vi "10-Tap 8-Bit Camera with DRAM (Host).vi"() -> ()   [LabVIEW 2018]
doc: "This is the host VI for the 10-Tap 8-Bit Camera with DRAM example. This example demonstrates how to acquire images from a 10-tap, 8-bit, extended configuration, Camera Link camera and display the images on the host. This example supports area scan and line scan cameras for both continuous and finite acquisitions.\n\nThis example also demonstrates the use of DRAM as a frame buffer for very high speed acquisitions. Data packing and flow-control are also employed to maximize use of the available DRAM and FIFOs in terms of both memory space and performance.\n\nAdditionally, the example demonstrates the serial server, which allows third-party camera configuration utilities to communicate with the camera using the Camera Link serial interface while this VI is running."
uses:
  <vilib>/userdefined/High Color/nirio_resource_hc.ctl
  <vilib>/Analysis/Matrix/Datatypes/RealMatrix.ctl
  <vilib>/Platform/TimedLoop/XDataNode/timing_clust.ctl
  <vilib>/Platform/TimedLoop/XDataNode/nitl_modes.ctl
  <vilib>/Platform/TimedLoop/XDataNode/wakeup.ctl
  <vilib>/DAQmx/write.llb/DAQmx Write (Analog DBL 1Chan 1Samp).vi
  <vilib>/Analysis/baseanly.llb/Real A x B.vi
  <vilib>/FPGAPlugInAG/PCIe-1473R/niLvFpga_Open_PCIe-1473R.vi
  <vilib>/rvi/interface/common/dynamic/niFpgaDynamicAddResources.vi
  <vilib>/FPGAPlugInAG/Dynamic/niLvFpga_Reset_Dynamic.vi
  <vilib>/Analysis/Matrix/Numeric/Conversions/Array To Matrix - RA2.vi
  <userlib>/DAQNavi Polymorphic VI/create/DAQNavi Create Channel(CI-UpDown Count Value).vi
  <vilib>/Utility/error.llb/Error Cluster From Error Code.vi
  <vilib>/rvi/errors/niLvFpgaAdjustHostInterfaceError.vi
  <vilib>/FPGAPlugInAG/Dynamic/niLvFpga_Run_Dynamic.vi
  <vilib>/rvi/interface/common/niFpgaWaitOnOcc.vi
  <userlib>/DAQNavi Polymorphic VI/read/DAQNavi Read (Counter Count Value 1Chan 1Samp).vi
  <vilib>/Analysis/Matrix/Numeric/Conversions/Array To Matrix - RA.vi
  <vilib>/Analysis/Matrix/Numeric/Conversions/Matrix To Array - RM.vi
  <vilib>/DAQmx/miscellaneous.llb/DAQmx Fill In Error Info.vi
  <vilib>/FPGAPlugInAG/Dynamic/niLvFpga_Close_Dynamic.vi
  <vilib>/platform/TimedLoop/XDataNode/XDataNode.xnode
  <vilib>/rvi/interface/nirviOpenFPGA/nirviOpenFPGA.xnode
  FPGA Bitfiles/10-Tap8-bitCamer_FPGATarget_10-Tap8-bitCamer_C490DC32.lvbitx
  <vilib>/rvi/interface/nirviMethod/nirviMethod.xnode
  <vilib>/rvi/interface/nirviReadWriteControl/nirviReadWriteControl.xnode
  <vilib>/rvi/interface/nirviCloseFPGA/nirviCloseFPGA.xnode
  <vilib>/rvi/interface/Simulation/niFpgaSimulationCallBeginRW.vi
  <vilib>/rvi/errors/niLvFpgaMergeErrorWithErrorCode.vi
  NiFpgaLv.dll
  <vilib>/FPGAPlugInAG/Dynamic/niLvFpga_ConfigureFifo_Dynamic.vi
  <vilib>/FPGAPlugInAG/Dynamic/niLvFpga_StartFifo_Dynamic.vi
  <vilib>/FPGAPlugInAG/Dynamic/niLvFpga_ReadFifo_Dynamic.vi
  <vilib>/Platform/TimedLoop/XDataNode/XDNodeRunTimeDep.lvlib
  <resource>/objmgr/ni.dex.rc
  MPC_dll_4_vs17_cv3_4/x64/Release/MPC_dll_4_vs17_cv3_4.dll
  <vilib>/ErrorRing/Error Ring.xnode
  <vilib>/Analysis/NI_AALBase.lvlib
  <vilib>/Analysis/Matrix/NI_Matrix.lvlib
  fish tracking dll vc17 opencv3_4/x64/Release/fish tracking dll vc17 opencv3_4.dll
panel:
  in  "length_fish":i32=115
  in  "width_fish":i32=20
  in  "ROI_height":i32=110
  in  "ROI_witdth":i32=110
  in  "Object Threshold":i32=200
  in  "BinThreshold":i32=100
  in  "Templates size":i32=48
  in  "shift_head2yolk":i32=30
  in  "address":string="192.168.1.27"
  out "# elements in queue 2":i32
  out "Numeric":i32
  out "concatenated string":string
  out "bytes written":i32
  in  "shift":i32=9
  in  "gamma":dbl=0.04 format="%#_13g"
  out "Cluster":cluster{"data":i32, i32}
  out "Real Matrix 5":T1
  out "Real Matrix 4":T1
  out "Real Matrix 2":T1
  out "Real Matrix":T1
  out "A x B 2":T1
  out "A x B":T1
  out "error out":errorcluster
  in  "send":bool
  out "Is Connected":bool
  in  "update ratio":dbl=0.1
  in  "Start Serial Server":bool=TRUE
  in  "Stopped 2":bool
  in  "display":bool
  out "Image":T2(plugin-control)
  in  "reset 2":bool
  in  "reset frame":bool
  in  "reset position":bool
  out "max load a frame":dbl
  out "max load a position":dbl
  out "# elements in queue":i32
  out "element":dbl[](array[numeric])
  in  "start sending":bool
  out "connected":bool
  in  "Acquire":bool
  out "max distance 2":i32
  out "out of FOV 2":i32
  in  "count":bool
  out "max distance":i32
  out "out of FOV":i32
  out "Stage Position Y":i32=520
  out "Stage Position X":i32=520
  out "#timeout3":i32
  out "#timeout1":i32
  out "max time4 image and position loading":dbl
  out "max time3 total":dbl
  out "max time2 detection":dbl
  out "max time1 detection+command":dbl
  out "time loading a frame":dbl
  in  "length of fish_history":i32=4
  in  "m(length of kernel)":i32=30
  out "Heading":cluster{dbl, dbl}
  out "process":i32
  in  "Target Y":i32(slide)=177 min=0 max=384 scale=130.0..230.0
  in  "Target X":i32(slide)=198 min=0 max=520 scale=130.0..230.0
  out "y":dbl
  out "x":dbl
  in  "Controller":picture
  out "Y Resolution":i32
  out "X Resolution":i32
  in  "Track":bool
  out "Frame #":i32=72
  out "电压2":dbl
  out "电压1":dbl
  out "fish FOUND":bool
  out "Centroid":cluster{"x":i32, "y":i32}
  out "TimeDelay":dbl
  in  "DMA Buffer Size\n(In Images)":u32=64 caption="DMA Buffer Size"
  in  "Signal Mapping":T3(ring)=enum."Basler 10-tap"
  out "Acq In Progress":bool
  in  "Line Scan":bool
  in  "Cancel":bool
  out "Acq'd Frame Width":u32
  in  "Stopped":bool
  in  "RIO Device":T4="RIO0"
  out "DMA Write Timeout":bool
  out "Frames Acq'd":u32
  out "Acq'd Frame Height":u32
  in  "Stop":bool
  in  "Image Height":u32=360 max=65535
  in  "Image Width":u32=360 max=65535 step=40
  out "Initialized":bool
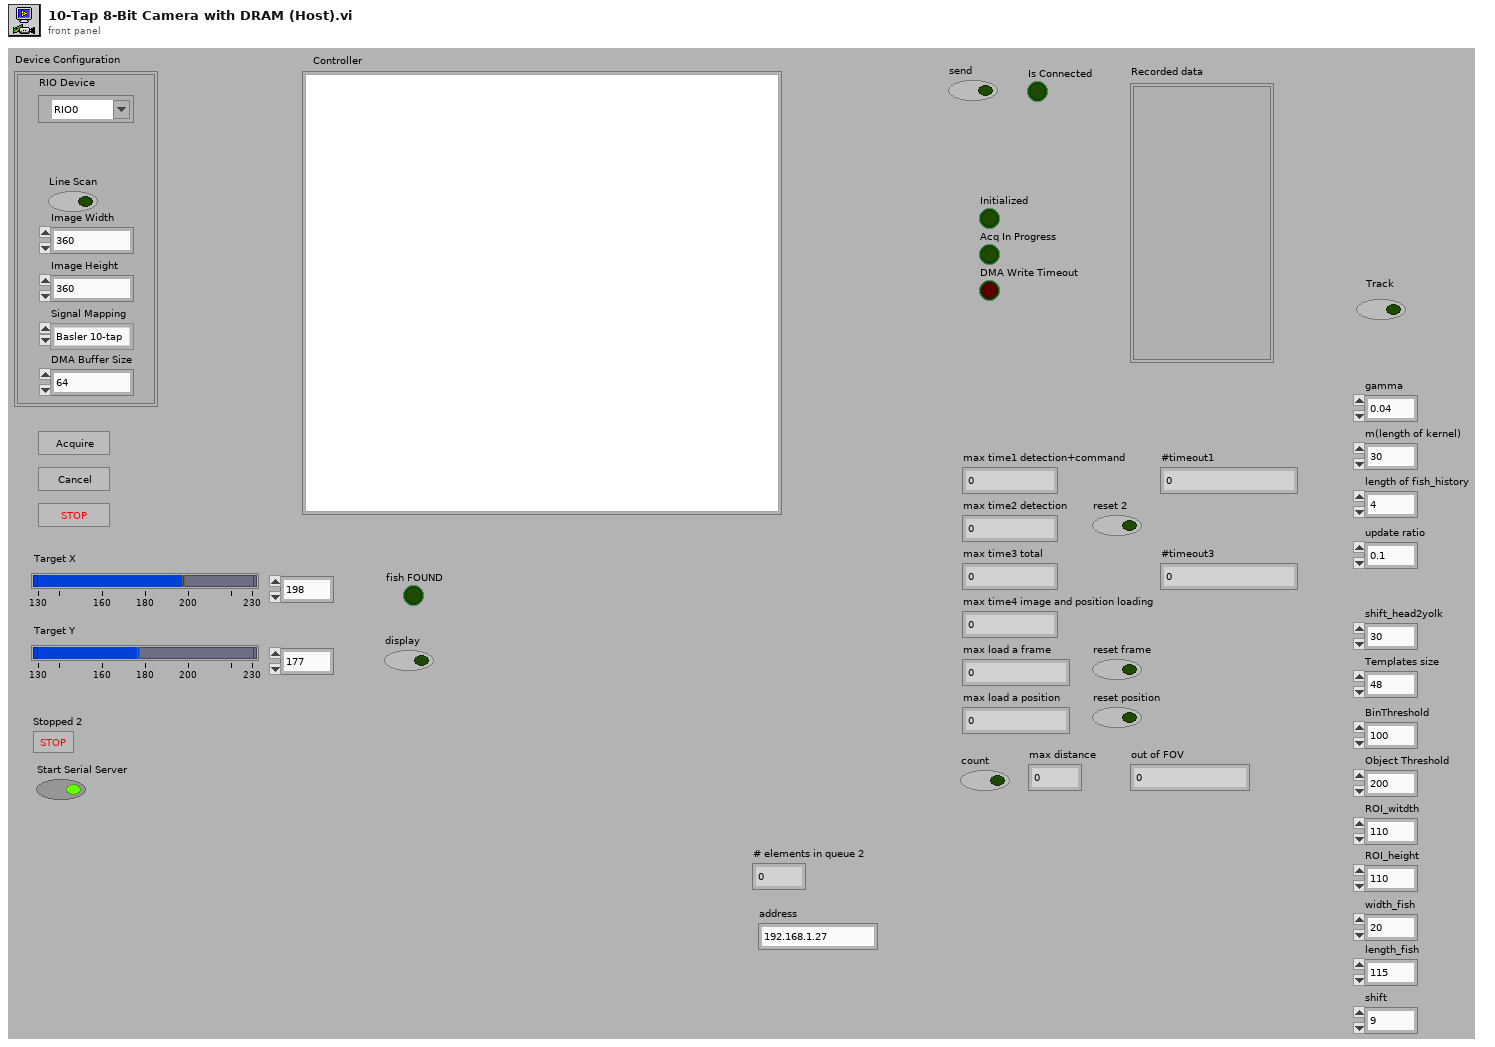
[diagram p1: front panel]
types:
  T1 = typedef "NI_Matrix.lvlib/RealMatrix.ctl" = dbl[][]
  T2 = typedef "IMAQ Image.ctl" = refnum<image>
  T3 = enum8{"Standard", "Basler 10-tap", "Vosskühler 10-tap"}
  T4 = typedef "nirio_resource_hc.ctl" = tag
  T5 = typedef "Image Type" = u32
  T6 = typedef "XDNodeRunTimeDep.lvlib/timing_clust.ctl" = cluster{"Expected End [f-1]":u64, "Actual End [f-1]":u64, "Finished Late? [f-1]":bool, "Expected End [i-1]":u64, "Actual End [i-1]":u64, "Finished Late? [i-1]":bool, "Expected Start [i]":u64, "Actual Start [i]":u64, "Expected Start [f]":u64, "Actual Start [f]":u64, "Source Name":string, "Structure Name":string, "Period":i64, "Deadline":i64, "Offset":i64, "Start":i64, "Priority":i32, "Timeout":i32, "Mode":T7, "Wakeup Reason":T8, "Error":errorcluster, "Source Type":string, "Secondary Source Type":string, "Global End Time":u64, "Global Start Time":u64, "Frame Duration":u64, "Iteration Duration":u64, "Assigned CPU":i32, "I/O Scan Engine Mode":u32}
  T7 = typedef "XDNodeRunTimeDep.lvlib/nitl_modes.ctl" = enum32{"No Change", "Process missed periods, maintain original phase", "Discard missed periods, maintain original phase", "Process missed periods, ignore original phase", "Discard missed periods, ignore original phase"}
  T8 = typedef "XDNodeRunTimeDep.lvlib/wakeup.ctl" = enum32{"Normal", "Aborted", "Asynchronous wakeup", "Timing source error", "Timed loop error", "Timeout"}
  T9 = enum16{"big-endian, network order", "native, host order", "little-endian"}
  T10 = typedef "LVPoint32TypeDef.ctl" = cluster{"Horizontal":i32, "Vertical":i32}
  T11 = typedef "LVPositionTypeDef.ctl" = cluster{"Left":i32, "Top":i32}
  T12 = typedef "LVBoundsTypeDef.ctl" = cluster{"Width":u32, "Height":u32}
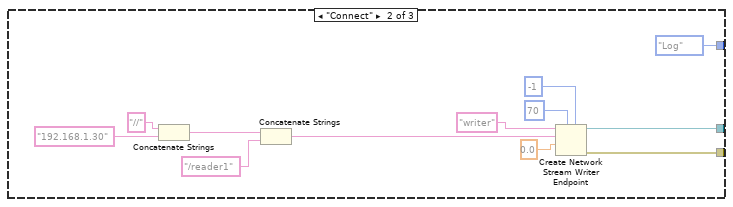
[diagram p4: hidden frame]
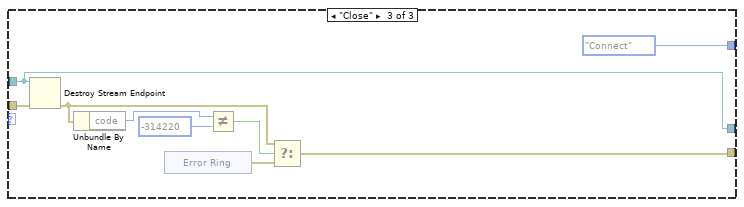
[diagram p5: hidden frame]
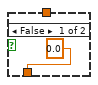
[diagram p13: hidden frame]
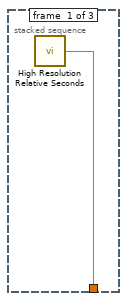
[diagram p14: hidden frame]
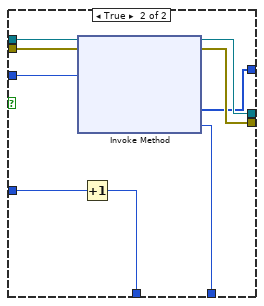
[diagram p15: hidden frame]
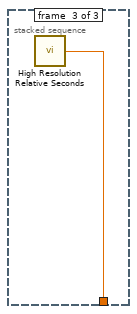
[diagram p16: hidden frame]
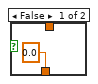
[diagram p17: hidden frame]
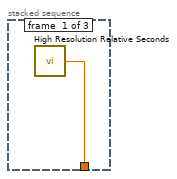
[diagram p18: hidden frame]
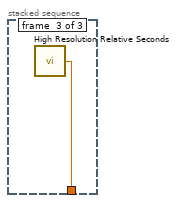
[diagram p19: hidden frame]
diagram:
  w38 = 72 ("n_templates")
  w40 = 0
  w61 = 2
  w55 = 0
  w62 = 0.0
  w86 = T5 0 items=["Grayscale (U8)", "Grayscale (I16)", "Grayscale (SGL)", "Complex (CSG)", "RGB (U32)", "HSL (U32)", "RGB (U64)", "Grayscale (U16)"] ("Image Type")
  w100 = refnum<k21> "Stage_Y"  # DAQmx任务名
  w101 = refnum<k21> "Stage_X"  # DAQmx任务名
  w103 = T5 0 items=["Grayscale (U8)", "Grayscale (I16)", "Grayscale (SGL)", "Complex (CSG)", "RGB (U32)", "HSL (U32)", "RGB (U64)", "Grayscale (U16)"] ("Image Type")
  w109 = u32 8  # Pixels per DMA word
  w140 = T5 0 items=["Grayscale (U8)", "Grayscale (I16)", "Grayscale (SGL)", "Complex (CSG)", "RGB (U32)", "HSL (U32)", "RGB (U64)", "Grayscale (U16)"] ("Image Type")
  # "Start the Serial Server to allow serial communication\nwith the camera. This allows third-party camera\nconfiguration utilites to be used."
  # "If your camera outputs active-low enable\nsignals or does not use DVAL then you \ncan change the configuration here."
  # "Configure the DMA FIFO memory buffer to be\nlarge enough for several frames. This provides\nbuffering to help deal with system latencies."
  # "Start running\nthe FPGA VI."
  # "Reset FPGA to clear\nany current state."
  # "Read the specified image\nwidth and height. In this\nexample, these must be set\nbefore starting the VI."
  # "Merge any errors.\nClean up the image.\nClose the FPGA reference.\nDisplay any errors."
  # "Acquire frames as requested.\nUse the width and height to determine how much data to read from the DMA FIFO.\nConvert the data into a Vision Image for display."
  # "Monitor the acquisition status"
  # "Create an image of the type to be displayed."
  # "Initialize the acquisition interface on the FPGA.  This will\nwait until a pixel clock is detected from the camera."
  # "Initialize the DMA FIFO for transferring\ndata from FPGA target to the host."
  # "Configure the Camera Link interface.\nThis needs to be done prior to running\nthe FPGA block diagram."
  # "Open a reference to the FPGA bitstream\nand initialize the user interface."
  n1 = flat-sequence {
    tunnel: [w146] -> w135
    tunnel: [w145] -> w144
    frame #0 {
      w149 = u32 0 ("Num Lines Acq'd")
      w148 = FALSE ("stop")
      n2 = local write "DMA Write Timeout"(w148) -> ()
      n3 = local write "Acq'd Frame Width"(w149) -> ()
      n4 = local write "Acq'd Frame Height"(w149) -> ()
      n5 = local write "Stopped"(w148) -> ()
      n6 = local write "Frames Acq'd"(w149) -> ()
      n7 = local write "Initialized"(w148) -> ()
      n8 = xnode "打开FPGA VI引用句柄"("resource name"="RIO Device") -> ("FPGA VI Reference Out"=w146:refnum<k20>, "error out"=w145:errorcluster)  [unwired: 1 in]
    }
  }
  n9 = xnode "Invoke Method"("FPGA VI Reference In"=w135, "error in"=w144) -> ("FPGA VI Reference Out"=w125:refnum<k20>, "error out"=w127:errorcluster)
  n10 = xnode "Read/Write Control"("FPGA VI Reference In"=w125, "error in"=w127, "CL Config.FVAL Active High"=TRUE ("IO Module Config.CL FVAL Active High"), "CL Config.LVAL Active High"=TRUE ("IO Module Config.CL LVAL Active High"), "CL Config.DVAL Active High"=TRUE ("IO Module Config.CL DVAL Active High"), "CL Config.Spare Active High"=TRUE ("IO Module Config.CL Spare Active High"), "CL Config.Line Scan"="Line Scan", "Acq Control.Ignore DVAL"=FALSE ("CL Config.Line Scan"), "CL Config.Configuration"=enum8{"Base", "Medium", "Full"}."Full", "CL Config.Signal Mapping"="Signal Mapping") -> ("FPGA VI Reference Out"=w128:refnum<k20>, "error out"=w126:errorcluster)
  n11 = xnode "Invoke Method"("FPGA VI Reference In"=w128, "error in"=w126) -> ("FPGA VI Reference Out"=w106:refnum<k20>, "error out"=w105:errorcluster)  [unwired: 1 in]
  n12 = Multiply(x="Image Height", y="Image Width") -> (x*y=w108:u32)
  n13 = Quotient & Remainder(x=w108, y=w109) -> (floor(x/y)=w107:u32)  [unwired: 1 out]
  n14 = Multiply(x=w107, y="DMA Buffer Size\n(In Images)") -> (x*y=w119:u32)
  n15 = xnode "Invoke Method"("FPGA VI Reference In"=w106, "error in"=w105, "请求的深度"=w119) -> ("FPGA VI Reference Out"=w134:refnum<k20>, "error out"=w133:errorcluster)  [unwired: 1 out]
  n16 = xnode "Invoke Method"("FPGA VI Reference In"=w134, "error in"=w133) -> ("FPGA VI Reference Out"=w120:refnum<k20>, "error out"=w132:errorcluster)
  n17 = xnode "读取/写入控件"("FPGA VI Reference In"=w120, "error in"=w132, "Acq Control.Initialize"=TRUE ("Arm Acquisition")) -> ("FPGA VI Reference Out"=w143:refnum<k20>, "error out"=w142:errorcluster)
  n18 = while {
    tunnel: w143 -> [w157]
    tunnel: w142 -> [w156]
    tunnel: [w155] -> w25
    tunnel: [w159] -> w116
    i -> [w151]
    stop <- w162 stop-if-true
    # "A custom error is generated if the acquisition unit has not become\ninitialized within 2 seconds. This typically occurs when a camera is\nnot connected, is not powered, or is not of the correct type."
    n19 = xnode "读取/写入控件"("FPGA VI Reference In"=w157, "error in"=w156) -> ("FPGA VI Reference Out"=w155:refnum<k20>, "error out"=w154:errorcluster, "Acq Status.Initialized"=w153:bool)
    n20 = Wait (ms)(milliseconds to wait=u32 100) -> ()  [unwired: 1 out]
    n21 = Greater?(x=w151, y=20) -> (0:w152:bool)
    n22 = case shown="True" w152 {
      tunnel: [w164 FALSE] -> w158
      tunnel: w153 -> [w164 _]
      tunnel: w154 -> [w163 w166]
      tunnel: [w163 w168] -> w159
      frame False {
      }
      frame True {
        n23 = Merge Errors(w166, errorcluster {"status"=TRUE, "code"=-8999, "source"="Acquisition Initialization: This error typically occurs when a camera is not properly connected, is not powered, or is not of the correct type."} ("error in")) -> (w168:errorcluster)
      }
    }
    "Initialized" <- w158
    n24 = Unbundle By Name(w159) -> ("status"=w161:bool)
    n25 = Or(x=w161, y=w158) -> (x .or. y?=w162:bool)
  }
  n26 = case shown="True" "Start Serial Server" {
    tunnel: [_ w169] -> w24
    tunnel: w25 -> [_ w170]
    frame False {
    }
    frame True {
      n27 = control-ref of="Stopped 2"() -> (w171:refnum<vi>)
      n28 = call "SerialServer.vi"("Stop Refnum"=w171, "FPGA VI Reference In"=w170) -> ("FPGA VI Reference Out"=w169:refnum<k20>)  [unwired: 5 in]
    }
  }
  n29 = call "IMAQ Create"("Image Name"="Image", "Image Type"=w140, "error in (no error)"=w116) -> ("New Image"=w113:T2, "error out"=w112:errorcluster)  [unwired: 2 in]
  n30 = Add(x="length of fish_history", y=1) -> (x+y=w57:i32)
  n31 = Initialize Array(0.0, 7) -> (w27:dbl[])
  n32 = Obtain Queue(max queue size (-1, unlimited)=3, name (unnamed)="tracking result" ("Image Name"), element data type=w27) -> (queue out=w23:refnum<queue>)  [unwired: 2 in, 2 out]
  n33 = Multiply(x=w61, y=w57) -> (x*y=w54:i32)
  n34 = To Unsigned Byte Integer(number=w40) -> (unsigned 8bit integer=w41:u8)
  n35 = Add(x="m(length of kernel)", y=1) -> (x+y=w42:i32)
  n36 = Initialize Array(w41, w40, w40, w40) -> (w39:u8[][][])
  n37 = for {
    N: w38 -> [_]
    shift-right: [w173] -> w37
    shift-left: w39 -> [w174]
    i -> [w172]
    w178 = T5 0 items=["Grayscale (U8)", "Grayscale (I16)", "Grayscale (SGL)", "Complex (CSG)", "RGB (U32)", "HSL (U32)", "RGB (U64)", "Grayscale (U16)"] ("Image Type")
    n38 = Number To Decimal String(number=w172) -> (decimal integer string=w182:string)  [unwired: 1 in]
    n39 = Concatenate Strings(w182, ".jpg") -> (w181:string)
    n40 = Build Path(base path=path "F:/TrackingUsingOpenCV3_with_bkg_subtr_and_pred_and_temp_matching_nodisplay - 210309/templates" ("Templates Path"), name or relative path=w181) -> (appended path=w180:path)
    n41 = call "IMAQ Create"("Image Name"="Temp", "Image Type"=w178) -> ("New Image"=w177:T2)  [unwired: 3 in, 1 out]
    n42 = call "IMAQ ReadFile"("File Path"=w180, "Image"=w177) -> ("Image Out"=w176:T2)  [unwired: 5 in, 4 out]
    n43 = call "IMAQ ImageToArray"("Image"=w176) -> ("Image Pixels (U8)"=w175:u8[][])  [unwired: 3 in, 4 out]
    n44 = Insert Into Array(array=w174, index (dim 0)=w172, new element=w175) -> (w173:u8[][][])  [unwired: 2 in]
  }
  n45 = Multiply(x=w61, y=w42) -> (x*y=w60:i32)
  n46 = Obtain Queue(max queue size (-1, unlimited)=w60, name (unnamed)="command_history", element data type=w62) -> (queue out=w64:refnum<queue>)  [unwired: 2 in, 2 out]
  n47 = Obtain Queue(max queue size (-1, unlimited)=w54, name (unnamed)="stage_position_history", element data type=w55) -> (queue out=w53:refnum<queue>)  [unwired: 2 in, 2 out]
  n48 = Obtain Queue(max queue size (-1, unlimited)=w54, name (unnamed)="fish_tr_history", element data type=w55) -> (queue out=w66:refnum<queue>)  [unwired: 2 in, 2 out]
  n49 = Obtain Queue(max queue size (-1, unlimited)=w54, name (unnamed)="fish_heading_history", element data type=w62) -> (queue out=w65:refnum<queue>)  [unwired: 2 in, 2 out]
  n50 = for "For循环" {
    N: w60 -> [_]
    tunnel: w64 -> [w187]
    tunnel: [w186] -> w63
    n51 = Lossy Enqueue Element(queue=w187, element=0.0) -> (queue out=w186:refnum<queue>)  [unwired: 1 in, 3 out]
  }
  n52 = TCP Open Connection(address="address", remote port or service name=u16 11000) -> (connection ID=w4:refnum<k5>, error out=w3:errorcluster)  [unwired: 3 in]
  n53 = call-poly <userlib>:"DAQNavi Create Channel.vi"("physical channels"="PCI-1784,BID#1/cntr0" ("Image Name"), "signal counting type"="AbPhaseX4" ("Image Name"), "initial value"="0" ("Image Name")) -> ("task out"=w81:i32)  [unwired: 11 in, 1 out]
  n54 = call-poly <userlib>:"DAQNavi Create Channel.vi"("physical channels"="PCI-1784,BID#1/cntr1" ("Image Name"), "signal counting type"="AbPhaseX4" ("Image Name"), "initial value"="0" ("Image Name")) -> ("task out"=w80:i32)  [unwired: 11 in, 1 out]
  n55 = node-c288() -> (w8:T6)  [unwired: 4 in]
  n56 = disable-structure shown="Disabled" {
    disable-tunnel: w23 -> [w191 _]
    frame Disabled {
      n57 = while "Target->Host Data Writer" {
        shift-right: [w199] -> w189
        shift-left: _ -> [w202]
        shift-right: [w198] -> _
        shift-left: _ -> [w203]
        shift-right: [w200] -> _
        shift-left: enum16{"Log", "Connect", "Close"}."Log" -> [w201]
        tunnel: w191 -> [w194]
        tunnel: [w193] -> w188
        stop <- w192 stop-if-true
        # "Send Data to Host VI"
        n58 = case shown="\"Log\", Default" w201 {
          tunnel: [w220 w227 w245] -> w198
          tunnel: w203 -> [w223 _ w245]
          tunnel: w202 -> [w222 _ w246]
          tunnel: [w221 w228 w239] -> w199
          tunnel: [w224 enum16{"Log", "Connect", "Close"}."Log" enum16{"Log", "Connect", "Close"}."Connect"] -> w200
          frame "Log", Default {
            (unwired) 0 ("timeout ms")
            n59 = property class="Network Stream Endpoint"(reference=w223, error in=w222) -> (reference out=w220:refnum<k21>, error out=w221:errorcluster, "Connected"=w219:bool)
            "Is Connected" <- w219
            n60 = Select(t=enum16{"Log", "Connect", "Close"}."Log", s=w219, f=enum16{"Log", "Connect", "Close"}."Close") -> (s? t:f=w224:enum16{"Log", "Connect", "Close"})
          }
          frame "Connect" {
            n61 = Concatenate Strings("//" ("reader url"), "192.168.1.30" ("Target IP Address")) -> (w233:string)
            n62 = Concatenate Strings(w233, "/reader1" ("reader url")) -> (w231:string)
            n63 = Create Network Stream Writer Endpoint(5:-1 ("timeout in ms (-1)"), 7:70, 9:0.0, 10:w231, 11:"writer") -> (0:w228:errorcluster, 3:w227:refnum<k21>)  [unwired: 2 in]
          }
          frame "Close" {
            n64 = Destroy Stream Endpoint(8:w246, 11:w245) -> (0:w240:errorcluster)
            n65 = Unbundle By Name(w240) -> ("code"=w244:i32)
            n66 = xnode "Error Ring"() -> ("error out"=w241:errorcluster)
            n67 = Not Equal?(x=w244, y=-314220) -> (x != y?=w242:bool)
            n68 = Select(t=w240, s=w242, f=w241) -> (s? t:f=w239:errorcluster)
          }
        }
        n69 = property class="Network Stream Endpoint"(reference=w198, error in=w199) -> (reference out=w196:refnum<k21>, error out=w195:errorcluster, "Connected"=w197:bool)
        n70 = case shown="True" w197 {
          tunnel: w196 -> [_ w208]
          tunnel: w195 -> [_ w209]
          tunnel: w194 -> [w204 w207]
          tunnel: [w204 w205] -> w193
          frame False {
          }
          frame True {
            n71 = Get Queue Status(queue=w207) -> (queue out=w211:refnum<queue>)  [unwired: 2 in, 7 out]
            n72 = Dequeue Element(queue=w211) -> (queue out=w205:refnum<queue>, element=w210:dbl[])  [unwired: 2 in, 2 out]
            n73 = case shown="True" "send" {
              tunnel: w210 -> [_ w216]
              tunnel: w209 -> [_ w215]
              tunnel: w208 -> [_ w214]
              frame False {
              }
              frame True {
                w217 = 0 ("timeout ms (-1)")
                n74 = shared-variable-write(w214, w215, w216, w217) -> (w213:refnum<k21>, w218:errorcluster)  [unwired: 1 out]
                n75 = Flush Stream(8:w218, 9:w217, 11:w213) -> (0:→"error out":errorcluster)  [unwired: 1 in, 2 out]
              }
            }
          }
        }
        n76 = local read "Stop"() -> (w192:bool)
      }
      n77 = call <vilib>:"Simple Error Handler.vi"("error in (no error)"=w189) -> ()  [unwired: 4 in, 5 out]
      n78 = Release Queue(queue=w188) -> ()  [unwired: 2 in, 3 out]
    }
    frame Enabled {
    }
  }
  n79 = call "IMAQ Create"("Image Name"="BkgImageOpenCV", "Image Type"=w86) -> ("New Image"=w88:T2)  [unwired: 3 in, 1 out]
  n80 = call <userlib>:"DAQNavi Start Task.vi"("task in"=w81) -> ("task out"=w77:i32)  [unwired: 9 in, 1 out]
  n81 = call <userlib>:"DAQNavi Start Task.vi"("task in"=w80) -> ("task out"=w76:i32)  [unwired: 9 in, 1 out]
  n82 = call "IMAQ ReadFile"("File Path"=path "F:/TrackingUsingOpenCV3_with_bkg_subtr_and_pred_and_temp_matching_nodisplay - 210309/fish tracking dll vc17 opencv3_4/bkg_global.png" ("Bkg Image Path"), "Image"=w88) -> ("Image Out"=w11:T2)  [unwired: 5 in, 4 out]
  n83 = disable-structure shown="Disabled" {
    disable-tunnel: w23 -> [w249 _]
    frame Disabled {
      n84 = Concatenate Strings("//" ("reader url"), "192.168.1.19" ("Target IP Address")) -> (w260:string)
      n85 = Concatenate Strings(w260, "/reader1" ("reader url")) -> (w258:string)
      n86 = Create Network Stream Writer Endpoint(7:70, 9:0.0, 10:w258, 11:"writer") -> (0:w263:errorcluster, 3:w265:refnum<k21>)  [unwired: 3 in]
      n87 = property class="Network Stream Endpoint"(reference=w265, error in=w263) -> (reference out=w256:refnum<k21>, error out=w255:errorcluster, "Connected"=→"connected":bool)
      n88 = node-c288() -> (w269:T6)  [unwired: 4 in]
      n89 = timed-loop {
        tunnel: w249 -> [w276]
        tunnel: w256 -> [w275]
        tunnel: w255 -> [w274]
        tunnel: [w273] -> w252
        tunnel: [w272] -> w251
        tunnel: [w271] -> w250
        timing: w269 -> [_]
        timing-out: [_] -> w268
        stop <- w270 stop-if-true
        n90 = node-c288() -> ()  [unwired: 1 in, 1 out]
        n91 = case shown="True" "start sending" {
          tunnel: w275 -> [w281 w294]
          tunnel: w274 -> [w280 w293]
          tunnel: w276 -> [w282 w284]
          tunnel: [w282 w292] -> w273
          tunnel: [w281 w287] -> w272
          tunnel: [w280 w286] -> w271
          frame False {
          }
          frame True {
            w288 = 0
            n92 = Get Queue Status(queue=w284) -> (queue out=w285:refnum<queue>, # elements in queue=w283:i32)  [unwired: 2 in, 6 out]
            n93 = disable-structure shown="Disabled" {
              disable-tunnel: w283 -> [w295 _]
              frame Disabled {
                "# elements in queue" <- w295
              }
              frame Enabled {
              }
            }
            n94 = Dequeue Element(queue=w285) -> (queue out=w292:refnum<queue>, element=w291:dbl[])  [unwired: 2 in, 2 out]
            n95 = disable-structure shown="Disabled" {
              disable-tunnel: w291 -> [w296 _]
              frame Disabled {
                "element" <- w296
              }
              frame Enabled {
              }
            }
            n96 = shared-variable-write(w294, w293, w291, w288) -> (w290:refnum<k21>, w289:errorcluster)  [unwired: 1 out]
            n97 = Flush Stream(8:w289, 9:w288, 11:w290) -> (0:w286:errorcluster, 3:w287:refnum<k21>)  [unwired: 1 in, 1 out]
          }
        }
        n98 = local read "Stop"() -> (w270:bool)
        n99 = node-c288() -> ()  [unwired: 1 in, 1 out]
      }
      n100 = node-c288(w268) -> ()  [unwired: 1 out]
      n101 = Release Queue(queue=w252) -> ()  [unwired: 2 in, 3 out]
      n102 = Flush Stream(8:w250, 11:w251) -> (0:w253:errorcluster, 3:w254:refnum<k21>)  [unwired: 2 in, 1 out]
      n103 = Destroy Stream Endpoint(8:w253, 11:w254) -> ()  [unwired: 1 out]
    }
    frame Enabled {
    }
  }
  n104 = call "IMAQ GetImageSize"("Image"=w11) -> ("Y Resolution"=w9:i32, "X Resolution"=w10:i32)  [unwired: 3 in, 1 out]
  n105 = call-poly <vilib>:"Array To Matrix.vi"("Real 2D Array"=dbl[][] [[1.506559, -0.036078], [0.030048, 1.495542]]) -> ("Real Matrix"=w19:T1)
  "Real Matrix 5" <- w19
  n106 = Initialize Array(0.0, 2) -> (w14:dbl[])
  n107 = call-poly <vilib>:"Array To Matrix.vi"("Real 2D Array"=dbl[][] [[1.506559, -0.036078, 0.0], [0.030048, 1.495542, 1.506559], [-12.463135, -1.547689, 1.0]]) -> ("Real Matrix"=w20:T1)
  "Real Matrix 4" <- w20
  n108 = call "IMAQ ImageToArray"("Image"=w11) -> ("Image Pixels (U8)"=w12:u8[][])  [unwired: 3 in, 4 out]
  n109 = Obtain Queue(max queue size (-1, unlimited)=1, name (unnamed)="stage postion" ("Image Name"), element data type=w14) -> (queue out=w13:refnum<queue>)  [unwired: 2 in, 2 out]
  n110 = timed-loop {
    tunnel: w4 -> [w320]
    tunnel: w3 -> [w319]
    timing: w8 -> [_]
    timing-out: [_] -> w7
    tunnel: [w313] -> w2
    tunnel: [w312] -> w1
    tunnel: w13 -> [w307]
    i -> [w309]
    stop <- w314 stop-if-true
    w311 = 6
    n111 = node-c288() -> ()  [unwired: 1 in, 1 out]
    n112 = Get Queue Status(queue=w307) -> (queue out=w308:refnum<queue>, # elements in queue=→"# elements in queue 2":i32)  [unwired: 2 in, 6 out]
    n113 = Dequeue Element(queue=w308) -> (element=w303:dbl[])  [unwired: 2 in, 3 out]
    n114 = Index Array(array=w303, index=0) -> (element=w302:dbl)
    n115 = Index Array(array=w303, index=1) -> (element=w300:dbl)
    n116 = Absolute Value(x=w302) -> (abs(x)=w301:dbl)
    n117 = Absolute Value(x=w300) -> (abs(x)=w299:dbl)
    n118 = Number To Decimal String(number=w301, width (-)=w311) -> (decimal integer string=w318:string)
    n119 = Number To Decimal String(number=w299, width (-)=w311) -> (decimal integer string=w317:string)
    n120 = Concatenate Strings(w318, w317) -> (w316:string)
    "concatenated string" <- w316
    n121 = TCP Write(connection ID=w320, data in=w316, error in (no error)=w319, 9:0) -> (connection ID out=w313:refnum<k5>, bytes written=→"bytes written":i32, error out=w312:errorcluster)
    n122 = local read "Stop"() -> (w314:bool)
    n123 = node-c288() -> ()  [unwired: 1 in, 1 out]
    "Numeric" <- w309
  }
  n124 = node-c288() -> (w32:T6)  [unwired: 4 in]
  n125 = call "IMAQ Create"("Image Name"="DstImageOpenCV", "Image Type"=w103) -> ("New Image"=w102:T2)  [unwired: 3 in, 1 out]
  n126 = while {
    tunnel: w25 -> [w333]
    tunnel: [w336] -> w129
    stop <- w335 stop-if-true
    w326 = u32 10  # Pixels per clock
    # "Update status indicators"
    n127 = Wait Until Next ms Multiple(millisecond multiple=u32 100) -> ()  [unwired: 1 out]
    n128 = xnode "Read/Write Control"("FPGA VI Reference In"=w333) -> ("error out"=w332:errorcluster, "Acq Status.Lines Per Frame"=w329:u32, "Acq Status.Frames Acq'd"=w331:u32, "Acq Status.Clocks Per Line"=w327:u32, "Acq Status.Acq In Progress"=→"Acq In Progress":bool, "Acq Status.DMA Write Timeout"=w324:bool)  [unwired: 1 in, 1 out]
    "DMA Write Timeout" <- w324
    n129 = Multiply(x=w327, y=w326) -> (x*y=w328:u32)
    n130 = disable-structure shown="Disabled" {
      disable-tunnel: w331 -> [w339 _]
      disable-tunnel: w329 -> [w338 _]
      disable-tunnel: w328 -> [w337 _]
      frame Disabled {
        "Acq'd Frame Height" <- w338
        "Frames Acq'd" <- w339
        "Acq'd Frame Width" <- w337
      }
      frame Enabled {
      }
    }
    n131 = local read "Stopped"() -> (w323:bool)
    n132 = Compound Arithmetic op=AND(w324, invert w323) -> (w325:bool)
    n133 = case shown="True" w325 {
      tunnel: w332 -> [w344 _]
      tunnel: [w344 errorcluster {"status"=TRUE, "code"=-8999, "source"="DMA Write Timeout: The write operation to the DMA FIFO on the FPGA timed out. This can be caused by the DMA FIFO not being started or the DMA FIFO overflowing. Make sure that Start is being called on the DMA FIFO. Also make sure that the host application is reading from the DMA FIFO fast enough to prevent it from overflowing."} ("error out")] -> w336
      frame False {
      }
      frame True {
      }
    }
    n134 = flat-sequence {
      tunnel: w336 -> [w343]
      tunnel: [w341] -> w335
      frame #0 {
        n135 = Unbundle By Name(w343) -> ("status"=w342:bool)
        n136 = Or(x=w342, y="Stopped") -> (x .or. y?=w341:bool)
        n137 = local write "Stopped"(w341) -> ()
      }
    }
  }
  n138 = node-c288(w7) -> ()  [unwired: 1 out]
  n139 = TCP Close Connection(connection ID=w2, error in (no error)=w1) -> ()  [unwired: 1 in, 2 out]
  n140 = Open/Create/Replace File(file path (use dialog)=path "G:/Time.txt" ("Folder"), operation (0:open)=4) -> (refnum out=w46:refnum<file>)  [unwired: 4 in, 2 out]
  n141 = call <vilib>:"DAQmx Start Task.vi"("task/channels in"=w100) -> ("task out"=w98:refnum<k21>)  [unwired: 13 in, 1 out]
  n142 = call <vilib>:"DAQmx Start Task.vi"("task/channels in"=w101) -> ("task out"=w99:refnum<k21>)  [unwired: 13 in, 1 out]
  n143 = timed-loop {
    tunnel: w25 -> [w476]
    tunnel: w112 -> [w475]
    tunnel: w107 -> [w372]
    tunnel: "Image Height" -> [w371]
    tunnel: "Image Width" -> [w480]
    tunnel: w113 -> [w479]
    tunnel: [w361] -> w130
    tunnel: [w478] -> w139
    tunnel: [w477] -> w137
    tunnel: w102 -> [w474]
    tunnel: w99 -> [w473]
    tunnel: w98 -> [w472]
    tunnel: [w471] -> w97
    tunnel: [w470] -> w96
    tunnel: w12 -> [w469]
    tunnel: w77 -> [w462]
    tunnel: w76 -> [w461]
    tunnel: [w460] -> w73
    tunnel: [w459] -> w72
    shift-right: [w465] -> _
    shift-left: u32 0 -> [w466]
    shift-right: [w463] -> _
    shift-left: cluster{"y":i32, "x":i32} {"y"=0, "x"=0} ("Centroid") -> [w464]
    tunnel: w63 -> [w458]
    tunnel: w66 -> [w457]
    tunnel: w65 -> [w456]
    tunnel: w53 -> [w455]
    tunnel: [w454] -> w52
    tunnel: [w453] -> w51
    tunnel: [w452] -> w50
    tunnel: [w451] -> w49
    tunnel: w46 -> [w449]
    tunnel: [w448] -> w45
    shift-right: [w447] -> _
    shift-left: _ -> [w446]
    tunnel: w38 -> [w445]
    tunnel: w37 -> [w444]
    tunnel: w23 -> [w443]
    timing: w32 -> [_]
    timing-out: [_] -> w31
    border: u32 0 -> [_]
    tunnel: w20 -> [w357]
    tunnel: w19 -> [w355]
    tunnel: w13 -> [w352]
    tunnel: w10 -> [w351]
    tunnel: w9 -> [w347]
    i -> [w450]
    stop <- w467 stop-if-true
    # "Read one frame\nfrom DMA FIFO"
    # "If we're in an acquisition, wait until\nwe have at least one frame to read."
    n144 = node-c288() -> ()  [unwired: 1 in, 1 out]
    n145 = stacked-sequence {
      tunnel: [_ w491 _] -> w478
      tunnel: w476 -> [_ w490 _]
      tunnel: w475 -> [_ w489 _]
      tunnel: [_ w488 _] -> w361
      tunnel: [_ w487 _] -> w442
      tunnel: w372 -> [_ w486 _]
      tunnel: w371 -> [_ w485 _]
      tunnel: [w484 _ _] -> w369
      tunnel: [_ _ w539] -> w370
      frame #0 {
        n146 = call <vilib>:"High Resolution Relative Seconds.vi"() -> ("relative seconds"=w484:dbl)
      }
      frame #1 {
        n147 = while {
          tunnel: [w497] -> w487
          tunnel: w486 -> [w494]
          shift-right: [w505] -> w491
          shift-left: w490 -> [w504]
          shift-right: [w498] -> w488
          shift-left: w489 -> [w503]
          tunnel: w485 -> [w492]
          stop <- w493 stop-if-true
          n148 = feedback #1() -> (w499:u32)
          n149 = while {
            tunnel: w504 -> [w535]
            tunnel: w503 -> [w534]
            tunnel: [w532] -> w502
            tunnel: [w533] -> w501
            tunnel: w499 -> [w538]
            tunnel: [w536] -> w495
            stop <- w537 stop-if-true
            n150 = xnode "Read/Write Control"("FPGA VI Reference In"=w535, "error in"=w534, "Acq Control.Cancel Acq"="Cancel") -> ("FPGA VI Reference Out"=w533:refnum<k20>, "error out"=w532:errorcluster, "Acq Status.Acq In Progress"=w531:bool, "Acq Status.Frames Acq'd"=w530:u32)
            n151 = Greater?(x=w530, y=w538) -> (0:w536:bool)
            n152 = Compound Arithmetic op=OR(invert w531, w536) -> (w537:bool)
          }
          n153 = case shown="False" w495 {
            tunnel: w494 -> [w517 w528]
            tunnel: [w512 w527] -> w505
            tunnel: w502 -> [w519 w526]
            tunnel: w501 -> [w518 w525]
            tunnel: [w506 w524] -> w500
            tunnel: w499 -> [w507 w523]
            tunnel: [w511 w522] -> w498
            tunnel: [_ w521] -> w497
            tunnel: [w517 w520] -> w496
            tunnel: w492 -> [w516 _]
            frame False {
              n154 = xnode "Read/Write Control"("FPGA VI Reference In"=w518, "error in"=w519, "Acq Control.Line Scan Height"=w516, "Acq Control.Frames To Acq"=u32 0 ("Frames To Acquire")) -> ("FPGA VI Reference Out"=w514:refnum<k20>, "error out"=w513:errorcluster)
              n155 = call "Rising Edge Detect.vi"("Input"="Acquire") -> ("Pulse"=w510:bool)  [unwired: 4 in]
              n156 = xnode "Read/Write Control"("FPGA VI Reference In"=w514, "error in"=w513, "Acq Control.Acquire"=w510) -> ("FPGA VI Reference Out"=w512:refnum<k20>, "error out"=w511:errorcluster)
              n157 = Select(t=u32 0, s="Acquire", f=w507) -> (s? t:f=w506:u32)
            }
            frame True {
              n158 = xnode "Invoke Method"("FPGA VI Reference In"=w525, "error in"=w526, "元素数量"=w528) -> ("FPGA VI Reference Out"=w527:refnum<k20>, "error out"=w522:errorcluster, "数据"=w521:u64[], "剩余元素"=w520:u32)  [unwired: 1 in]
              n159 = Increment(x=w523) -> (x+1=w524:u32)
            }
          }
          n160 = feedback-in #1(w500) -> ()
          n161 = Less?(x=w496, y=w494) -> (x < y?=w493:bool)
        }
      }
      frame #2 {
        n162 = call <vilib>:"High Resolution Relative Seconds.vi"() -> ("relative seconds"=w539:dbl)
      }
    }
    n163 = disable-structure shown="Disabled" {
      disable-tunnel: w450 -> [w481 _]
      frame Disabled {
        "process" <- w481
      }
      frame Enabled {
      }
    }
    n164 = Not(x="reset frame") -> (.not. x?=w360:bool)
    n165 = Boolean To (0,1)(Boolean=w360) -> (0, 1=w365:i16)
    n166 = Subtract(x=w370, y=w369) -> (x-y=w366:dbl)
    n167 = feedback #2(-inf) -> (w368:dbl)
    n168 = Max & Min(x=w366, y=w368) -> (max(x,y)=w363:dbl)  [unwired: 1 out]
    n169 = Multiply(x=w363, y=w365) -> (x*y=w362:dbl)
    n170 = feedback-in #2(w362) -> ()
    n171 = case shown="True" w360 {
      tunnel: w363 -> [_ w483]
      tunnel: [0.0 w483] -> w359
      frame False {
      }
      frame True {
      }
    }
    "max load a frame" <- w359
    n172 = flat-sequence {
      tunnel: w446 -> [w564]
      tunnel: w455 -> [w565]
      tunnel: w456 -> [w566]
      tunnel: w457 -> [w567]
      tunnel: w458 -> [w568]
      tunnel: w461 -> [w562]
      tunnel: w462 -> [w563]
      tunnel: w464 -> [w569]
      tunnel: w466 -> [w570]
      tunnel: w469 -> [w571]
      tunnel: w474 -> [w572]
      tunnel: w442 -> [w573]
      tunnel: w479 -> [w574]
      tunnel: w480 -> [w575]
      tunnel: w371 -> [w576]
      tunnel: [w576] -> w441
      tunnel: [w575] -> w440
      tunnel: [w574] -> w439
      tunnel: [w573] -> w438
      tunnel: [w572] -> w437
      tunnel: [w571] -> w436
      tunnel: [w570] -> w435
      tunnel: [w569] -> w434
      tunnel: [w568] -> w433
      tunnel: [w567] -> w432
      tunnel: [w566] -> w431
      tunnel: [w565] -> w430
      tunnel: [w564] -> w429
      tunnel: [w561] -> w428
      tunnel: [w560] -> w427
      tunnel: [w559] -> w426
      tunnel: [w558] -> w425
      tunnel: w445 -> [w558]
      tunnel: [w557] -> w424
      tunnel: w444 -> [w557]
      tunnel: w443 -> [w556]
      tunnel: [w556] -> w423
      tunnel: w357 -> [w544]
      tunnel: [w544] -> w356
      tunnel: w355 -> [w543]
      tunnel: [w543] -> w353
      tunnel: w352 -> [w542]
      tunnel: w351 -> [w541]
      tunnel: [w541] -> w349
      tunnel: [w540] -> w348
      tunnel: w347 -> [w540]
      tunnel: [w625] -> w422
      tunnel: [w624] -> w421
      tunnel: [w623] -> w420
      tunnel: [w622] -> w419
      tunnel: [w621] -> w418
      tunnel: [w620] -> w417
      tunnel: [w619] -> w416
      tunnel: [w618] -> w415
      tunnel: [w600] -> w414
      tunnel: [w598] -> w413
      tunnel: [w617] -> w412
      tunnel: [w616] -> w411
      tunnel: [w615] -> w410
      tunnel: [w614] -> w409
      tunnel: [w610] -> w408
      tunnel: [w599] -> w407
      tunnel: w441 -> [w625]
      tunnel: w440 -> [w624]
      tunnel: w439 -> [w623]
      tunnel: w438 -> [w622]
      tunnel: w437 -> [w621]
      tunnel: w436 -> [w620]
      tunnel: w435 -> [w619]
      tunnel: w434 -> [w618]
      tunnel: w433 -> [w617]
      tunnel: w432 -> [w616]
      tunnel: w431 -> [w615]
      tunnel: w430 -> [w614]
      tunnel: w429 -> [w608]
      tunnel: w428 -> [w600]
      tunnel: w427 -> [w599]
      tunnel: w426 -> [w598]
      tunnel: [w597] -> w406
      tunnel: w425 -> [w597]
      tunnel: [w596] -> w405
      tunnel: w424 -> [w596]
      tunnel: [w595] -> w404
      tunnel: w423 -> [w595]
      tunnel: [w594] -> w358
      tunnel: w356 -> [w594]
      tunnel: [w593] -> w354
      tunnel: w353 -> [w593]
      tunnel: [w592] -> w350
      tunnel: w349 -> [w592]
      tunnel: w348 -> [w591]
      tunnel: [w591] -> w346
      tunnel: w450 -> [w683]
      tunnel: w449 -> [w682]
      tunnel: [w681] -> w448
      tunnel: w422 -> [w722]
      tunnel: w421 -> [w721]
      tunnel: w420 -> [w720]
      tunnel: w419 -> [w718]
      tunnel: w418 -> [w660]
      tunnel: w417 -> [w627]
      tunnel: w416 -> [w700]
      tunnel: w415 -> [w658]
      tunnel: w414 -> [w676]
      tunnel: w413 -> [w675]
      tunnel: w412 -> [w694]
      tunnel: w411 -> [w693]
      tunnel: w410 -> [w692]
      tunnel: w409 -> [w691]
      tunnel: w408 -> [w679]
      tunnel: [w631] -> w403
      tunnel: [w699] -> w402
      tunnel: [w676] -> w401
      tunnel: [w675] -> w400
      tunnel: [w665] -> w399
      tunnel: [w690] -> w398
      tunnel: [w689] -> w397
      tunnel: [w688] -> w396
      tunnel: [w687] -> w395
      tunnel: [w678] -> w394
      tunnel: [w677] -> w393
      tunnel: w407 -> [w634]
      tunnel: w406 -> [w673]
      tunnel: w405 -> [w671]
      tunnel: w404 -> [w666]
      tunnel: w358 -> [w647]
      tunnel: w354 -> [w646]
      tunnel: w350 -> [w629]
      tunnel: w346 -> [w628]
      tunnel: w403 -> [w967]
      tunnel: [w967] -> w392
      tunnel: w402 -> [w966]
      tunnel: [w966] -> w391
      tunnel: w401 -> [w965]
      tunnel: [w965] -> w390
      tunnel: w400 -> [w964]
      tunnel: [w964] -> w389
      tunnel: w399 -> [w963]
      tunnel: [w963] -> w388
      tunnel: w398 -> [w962]
      tunnel: [w962] -> w387
      tunnel: w397 -> [w961]
      tunnel: [w961] -> w386
      tunnel: w396 -> [w960]
      tunnel: [w960] -> w385
      tunnel: w395 -> [w959]
      tunnel: [w959] -> w384
      tunnel: w394 -> [w958]
      tunnel: [w958] -> w383
      tunnel: w393 -> [w957]
      tunnel: [w957] -> w382
      tunnel: w392 -> [w983]
      tunnel: w391 -> [w982]
      tunnel: w390 -> [w981]
      tunnel: w389 -> [w980]
      tunnel: w388 -> [w979]
      tunnel: w387 -> [w978]
      tunnel: w386 -> [w977]
      tunnel: w385 -> [w976]
      tunnel: w384 -> [w975]
      tunnel: [w974] -> w470
      tunnel: [w973] -> w471
      tunnel: w473 -> [w972]
      tunnel: w472 -> [w971]
      tunnel: w383 -> [w970]
      tunnel: w382 -> [w969]
      tunnel: [w983] -> w381
      tunnel: [w982] -> w380
      tunnel: [w981] -> w379
      tunnel: [w980] -> w378
      tunnel: [w979] -> w377
      tunnel: [w978] -> w376
      tunnel: [w977] -> w375
      tunnel: [w976] -> w374
      tunnel: [w975] -> w373
      tunnel: [w985] -> w451
      tunnel: [w986] -> w452
      tunnel: [w987] -> w453
      tunnel: [w988] -> w454
      tunnel: [w989] -> w463
      tunnel: [w990] -> w459
      tunnel: [w991] -> w460
      tunnel: [w992] -> w465
      tunnel: [w993] -> w477
      tunnel: w381 -> [w993]
      tunnel: w380 -> [w992]
      tunnel: w379 -> [w991]
      tunnel: w378 -> [w990]
      tunnel: w377 -> [w989]
      tunnel: w376 -> [w988]
      tunnel: w375 -> [w987]
      tunnel: w374 -> [w986]
      tunnel: w373 -> [w985]
      tunnel: [w984] -> w447
      frame #0 {
        n173 = stacked-sequence {
          tunnel: w563 -> [_ w589 _]
          tunnel: w562 -> [_ w588 _]
          tunnel: [_ w587 _] -> w561
          tunnel: [_ w586 _] -> w560
          tunnel: [_ w585 _] -> w559
          tunnel: [w579 _ _] -> w555
          tunnel: [_ _ w590] -> w554
          tunnel: w542 -> [_ w583 _]
          frame #0 {
            n174 = call <vilib>:"High Resolution Relative Seconds.vi"() -> ("relative seconds"=w579:dbl)
          }
          frame #1 {
            n175 = call-poly <userlib>:"DAQNavi Read.vi"("task in"=w588) -> ("data"=w584:i32, "task out"=w585:i32)  [unwired: 8 in, 1 out]
            n176 = call-poly <userlib>:"DAQNavi Read.vi"("task in"=w589) -> ("data"=w582:i32, "task out"=w587:i32)  [unwired: 8 in, 1 out]
            "Stage Position X" <- w582
            n177 = Negate(x=w584) -> (-x=w581:i32)
            "Stage Position Y" <- w581
            n178 = Build Array(w582, w581) -> (w580:i32[])
            n179 = Bundle("data"=w582, w581) -> (w586:cluster{"data":i32, i32})  [unwired: 1 in]
            n180 = Lossy Enqueue Element(queue=w583, element=w580) -> ()  [unwired: 1 in, 4 out]
          }
          frame #2 {
            n181 = call <vilib>:"High Resolution Relative Seconds.vi"() -> ("relative seconds"=w590:dbl)
          }
        }
        n182 = Not(x="reset position") -> (.not. x?=w547:bool)
        n183 = Boolean To (0,1)(Boolean=w547) -> (0, 1=w549:i16)
        n184 = Subtract(x=w554, y=w555) -> (x-y=w551:dbl)
        n185 = feedback #3(-inf) -> (w553:dbl)
        n186 = Max & Min(x=w551, y=w553) -> (max(x,y)=w546:dbl)  [unwired: 1 out]
        n187 = Multiply(x=w546, y=w549) -> (x*y=w548:dbl)
        n188 = feedback-in #3(w548) -> ()
        n189 = case shown="True" w547 {
          tunnel: w546 -> [_ w578]
          tunnel: [0.0 w578] -> w545
          frame False {
          }
          frame True {
          }
        }
        "max load a position" <- w545
      }
      frame #1 {
        n190 = call <vilib>:"High Resolution Relative Seconds.vi"() -> ("relative seconds"=w610:dbl)
        n191 = feedback #4() -> (w611:dbl)  [unwired: 1 in]
        n192 = feedback-in #4(w610) -> ()
        n193 = Subtract(x=w610, y=w611) -> (x-y=w613:dbl)
        "TimeDelay" <- w613
        n194 = Greater?(x=w613, y=0.0045) -> (0:w605:bool)
        n195 = Subtract(x=w610, y=w608) -> (x-y=→"time loading a frame":dbl)
        n196 = Select(t=1, s=w605, f=0) -> (s? t:f=w602:i32)
        n197 = feedback #5(0) -> (w603:i32)
        n198 = Add(x=w602, y=w603) -> (x+y=w601:i32)
        "#timeout3" <- w601
        n199 = feedback-in #5(w601) -> ()
      }
      frame #2 {
        w626 = 0
        w707 = 30.0 ("pixel/mm")
        w695 = 0.0
        # "Convert U64 array\nto U8 array"
        # "Convert array to\nimage for display"
        n200 = Add(x=1, y=w700) -> (x+y=w699:u32)
        n201 = Flatten To String(anything=w718, prepend array or string size? (T)=FALSE, byte order (0:big-endian, network order)=T9."native, host order") -> (data string=w716:string)  [unwired: 1 in, 2 out]
        n202 = disable-structure shown="Disabled" {
          disable-tunnel: w699 -> [w724 _]
          frame Disabled {
            "Frame #" <- w724
          }
          frame Enabled {
          }
        }
        n203 = String To Byte Array(string=w716) -> (unsigned byte array=w715:u8[])
        n204 = Reshape Array(w715, w722, w721) -> (w719:u8[][])
        n205 = call "IMAQ ArrayToImage"("Image Pixels (U8)"=w719, "Image"=w720) -> ("Image Out"=w631:T2)  [unwired: 8 in, 1 out]
        n206 = expression code="atan(x)"(-0.043 ("tan(theta)")) -> (w701:dbl)
        n207 = Divide(x=w707, y=10000.0) -> (x/y=w704:dbl)
        n208 = Divide(x=w707, y=12800.0) -> (x/y=w703:dbl)
        n209 = call "IMAQ GetImageSize"("Image"=w631) -> ("Y Resolution"=w667:i32, "X Resolution"=w668:i32)  [unwired: 3 in, 1 out]
        "X Resolution" <- w668
        "Y Resolution" <- w667
        n210 = call "IMAQ ImageToArray"("Image"=w631) -> ("Image Pixels (U8)"=w630:u8[][])  [unwired: 3 in, 4 out]
        n211 = disable-structure shown="Disabled" {
          disable-tunnel: w634 -> [w723 _]
          frame Disabled {
            "Cluster" <- w723
          }
          frame Enabled {
          }
        }
        n212 = call "IMAQ SetImageSize"("Y Resolution"=w667, "X Resolution"=w668, "Image"=w660) -> ("Image Out"=w633:T2)  [unwired: 2 in, 1 out]
        n213 = Bundle(w695, w695) -> (w670:cluster{dbl, dbl})  [unwired: 1 in]
        n214 = call "IMAQ ImageToArray"("Image"=w633) -> ("Image Pixels (U8)"=w632:u8[][])  [unwired: 3 in, 4 out]
        n215 = dll-call lib="F:/TrackingUsingOpenCV3_with_bkg_subtr_and_pred_and_temp_matching_nodisplay - 210309/fish tracking dll vc17 opencv3_4/x64/Release/fish tracking dll vc17 opencv3_4.dll" fn="?find_centroid@@YAHPEAEH0H0HHHHH0HHPEAV?$Point_@H@cv@@NNNHHHHHHH11PEAV?$Point_@N@2@N@Z"("ImagePtrSrc"=w630, "LineWidthSrc"=w626, "ImagePtrDst"=w632, "LineWidthDst"=w626, "ImagePtrBkg"=w627, "LineWidthBkg"=w626, "Width"=w668, "Height"=w667, "BkgWidth"=w629, "BkgHeight"=w628, "templates"=w671, "n_templates"=w673, "TemplatesSize"="Templates size", "position"=w634, "scale_x"=w704, "scale_y"=w703, "theta"=w701, "BinThreshold"="BinThreshold", "counting_threshold"="Object Threshold", "ROI_witdth"="ROI_witdth", "ROI_height"="ROI_height", "width_fish"="width_fish", "length_fish"="length_fish", "shift"="shift", "centroid_in"=w658, "centroid_out"=w658, "heading_vector"=w670, "Update_Ratio_Bkg"="update ratio") -> ("return type"=w698:i32, "centroid_out"=w665:cluster{"y":i32, "x":i32}, "heading_vector"=w664:cluster{dbl, dbl})  [unwired: 29 in, 2 out]
        "Centroid" <- w665
        "Heading" <- w664
        n216 = Quotient & Remainder(x=w683, y=2) -> (x-y*floor(x/y)=w685:i32)  [unwired: 1 out]
        n217 = Equal To 0?(x=w698) -> (x = 0?=w669:bool)
        "fish FOUND" <- w669
        n218 = Equal?(x=w685, y=0) -> (x = y?=w656:bool)
        n219 = Unbundle(w634) -> ("data"=w663:i32, w662:i32)
        n220 = Unbundle(w664) -> (w639:dbl, w638:dbl)
        n221 = Build Array(w639, w638) -> (w637:dbl[])
        n222 = call-poly <vilib>:"Array To Matrix.vi"("Real 1D Array"=w637) -> ("Real Matrix (Column Vector)"=w636:T1)
        n223 = Transpose Matrix(1:w636) -> (0:w635:T1)
        "Real Matrix 2" <- w635
        n224 = Unbundle(w665) -> ("y"=w645:i32, "x"=w644:i32)
        n225 = Build Array(w645, w644, 1) -> (w642:i32[])
        n226 = call-poly <vilib>:"Array To Matrix.vi"("Real 1D Array"=w642) -> ("Real Matrix (Column Vector)"=w641:T1)
        n227 = Transpose Matrix(1:w641) -> (0:w640:T1)
        "Real Matrix" <- w640
        n228 = call-poly <vilib>:"A x B.vi"("B"=w647, "A"=w640) -> ("A x B"=w655:T1)  [unwired: 1 out]
        "A x B" <- w655
        n229 = call-poly <vilib>:"A x B.vi"("B"=w646, "A"=w635) -> ("A x B"=w650:T1)  [unwired: 1 out]
        "A x B 2" <- w650
        n230 = call-poly <vilib>:"Matrix To Array.vi"("Real Matrix"=w655) -> ("Real 2D Array"=w654:dbl[][])
        n231 = call-poly <vilib>:"Matrix To Array.vi"("Real Matrix"=w650) -> ("Real 2D Array"=w652:dbl[][])
        n232 = Reshape Array(w654, 2) -> (w649:dbl[])
        n233 = Reshape Array(w652, 2) -> (w648:dbl[])
        n234 = Build Array (concatenate)(w663, w662, w649, w648) -> (w661:dbl[])
        n235 = case shown="True" w656 {
          tunnel: [w725 w729] -> w680
          tunnel: w666 -> [_ w731]
          tunnel: w661 -> [_ w730]
          tunnel: w660 -> [_ w727]
          frame False {
            n236 = call <vilib>:"High Resolution Relative Seconds.vi"() -> ("relative seconds"=w725:dbl)
          }
          frame True {
            n237 = call <vilib>:"High Resolution Relative Seconds.vi"() -> ("relative seconds"=w729:dbl)
            n238 = Build Array (concatenate)(w729, w730) -> (w728:dbl[])
            n239 = case shown="True" "display" {
              tunnel: w727 -> [_ w732]
              frame False {
              }
              frame True {
                n240 = disable-structure shown="Disabled" {
                  disable-tunnel: w732 -> [w733 _]
                  frame Disabled {
                    "Image" <- w733
                  }
                  frame Enabled {
                  }
                }
              }
            }
            n241 = Lossy Enqueue Element(queue=w731, element=w728) -> ()  [unwired: 1 in, 4 out]
          }
        }
        n242 = And(x=w669, y="Track") -> (x .and. y?=w659:bool)
        n243 = case shown="True" w659 {
          tunnel: [w745 w804] -> w678
          tunnel: [w746 w805] -> w677
          tunnel: w694 -> [w736 w869]
          tunnel: w693 -> [w743 w868]
          tunnel: w692 -> [w741 w867]
          tunnel: w645 -> [_ w790]
          tunnel: w644 -> [_ w791]
          tunnel: w639 -> [_ w859]
          tunnel: w638 -> [_ w858]
          tunnel: w691 -> [w739 w852]
          tunnel: w663 -> [_ w850]
          tunnel: w662 -> [_ w849]
          tunnel: [w737 w830] -> w690
          tunnel: [w738 w835] -> w689
          tunnel: [w742 w834] -> w688
          tunnel: [w740 w833] -> w687
          tunnel: w679 -> [_ w810]
          tunnel: w682 -> [w744 w809]
          tunnel: [w744 w808] -> w681
          tunnel: w680 -> [_ w806]
          frame False {
            n244 = event shown="[1] \"Controller\": Mouse Down" {
              selector: _ -> [_ _ _]
              dyn-events: _ -> [_ _ _]
              timeout: 1 -> [_ _ _]
              event "Controller": Mouse Up {
                n245 = event-data() -> ()  [unwired: 1 in, 8 out]
                n246 = local write "x"(0.0) -> ()
                n247 = local write "y"(0.0) -> ()
              }
              event "Controller": Mouse Down {
                n248 = event-data() -> ("Coords"=w773:T10)  [unwired: 1 in, 7 out]
                n249 = property on="Controller" class="Pict"() -> ("Position"=w772:T11, "Bounds"=w767:T12)  [unwired: 2 in, 2 out]
                n250 = Unbundle By Name(w773) -> ("Horizontal"=w771:i32, "Vertical"=w769:i32)
                n251 = Unbundle By Name(w767) -> ("Width"=w765:u32, "Height"=w761:u32)
                n252 = Unbundle By Name(w772) -> ("Left"=w770:i32, "Top"=w768:i32)
                n253 = Subtract(x=w769, y=w768) -> (x-y=w762:i32)
                n254 = Subtract(x=w771, y=w770) -> (x-y=w766:i32)
                n255 = Divide(x=w762, y=w761) -> (x/y=w754:dbl)
                n256 = Divide(x=w766, y=w765) -> (x/y=w764:dbl)
                n257 = Subtract(x=w754, y=0.5) -> (x-y=w757:dbl)
                n258 = Subtract(x=w764, y=0.5) -> (x-y=w758:dbl)
                n259 = Multiply(x=w758, y=-2.0) -> (x*y=→"x":dbl)
                n260 = Multiply(x=w757, y=-2.0) -> (x*y=→"y":dbl)
              }
              event Timeout {
                n261 = event-data() -> ()  [unwired: 1 in, 3 out]
              }
            }
            n262 = Get Queue Status(queue=w736) -> (queue out=w735:refnum<queue>, max queue size=w734:i32)  [unwired: 2 in, 6 out]
            n263 = for "For循环" {
              N: w734 -> [_]
              tunnel: w735 -> [w750]
              tunnel: [w749] -> w737
              n264 = Lossy Enqueue Element(queue=w750, element=0.0) -> (queue out=w749:refnum<queue>)  [unwired: 1 in, 3 out]
            }
            n265 = Flush Queue(queue=w743) -> (queue out=w742:refnum<queue>)  [unwired: 1 in, 2 out]
            n266 = Flush Queue(queue=w741) -> (queue out=w740:refnum<queue>)  [unwired: 1 in, 2 out]
            n267 = Flush Queue(queue=w739) -> (queue out=w738:refnum<queue>)  [unwired: 1 in, 2 out]
            n268 = local read "y"() -> (w746:dbl)
            n269 = local read "x"() -> (w745:dbl)
          }
          frame True {
            w795 = 0
            w802 = 23
            w815 = 0.0
            w824 = 2
            w828 = TRUE
            w840 = 1.0
            n270 = local read "Target Y"() -> (w792:i32)
            n271 = Subtract(x=w791, y=w792) -> (x-y=w786:i32)
            n272 = Absolute Value(x=w786) -> (abs(x)=w785:i32)
            n273 = Bundle("Target X"="Target X", "Target Y"="Target Y") -> (w811:cluster{"Target X":i32, "Target Y":i32})  [unwired: 1 in]
            n274 = Greater?(x=w785, y=w802) -> (0:w800:bool)
            n275 = local read "Target X"() -> (w789:i32)
            n276 = Get Queue Status(queue=w869, return elements? (F)=w828) -> (queue out=w831:refnum<queue>, elements=w819:dbl[])  [unwired: 1 in, 6 out]
            n277 = Subtract(x=w790, y=w789) -> (x-y=w784:i32)
            n278 = Get Queue Status(queue=w868) -> (queue out=w863:refnum<queue>, max queue size=w822:i32, # elements in queue=w864:i32)  [unwired: 2 in, 5 out]
            n279 = Equal?(x=w864, y=0) -> (x = y?=w865:bool)
            n280 = Absolute Value(x=w784) -> (abs(x)=w783:i32)
            n281 = Quotient & Remainder(x=w822, y=2) -> (floor(x/y)=w820:i32)  [unwired: 1 out]
            n282 = case shown="True" w865 {
              tunnel: w863 -> [w946 w949]
              tunnel: w790 -> [w945 w950]
              tunnel: w820 -> [_ w951]
              tunnel: [w942 w948] -> w862
              tunnel: w791 -> [w944 w947]
              frame False {
                n283 = Lossy Enqueue Element(queue=w946, element=w945) -> (queue out=w943:refnum<queue>)  [unwired: 1 in, 3 out]
                n284 = Lossy Enqueue Element(queue=w943, element=w944) -> (queue out=w942:refnum<queue>)  [unwired: 1 in, 3 out]
              }
              frame True {
                n285 = for "For循环" {
                  N: w951 -> [_]
                  tunnel: w950 -> [w956]
                  tunnel: w949 -> [w955]
                  tunnel: [w952] -> w948
                  tunnel: w947 -> [w953]
                  n286 = Lossy Enqueue Element(queue=w955, element=w956) -> (queue out=w954:refnum<queue>)  [unwired: 1 in, 3 out]
                  n287 = Lossy Enqueue Element(queue=w954, element=w953) -> (queue out=w952:refnum<queue>)  [unwired: 1 in, 3 out]
                }
              }
            }
            n288 = Get Queue Status(queue=w862, return elements? (F)=w828) -> (queue out=w834:refnum<queue>, elements=w829:i32[])  [unwired: 1 in, 6 out]
            n289 = Greater?(x=w783, y=w802) -> (0:w801:bool)
            n290 = Or(x=w800, y=w801) -> (x .or. y?=w799:bool)
            n291 = Get Queue Status(queue=w867) -> (queue out=w856:refnum<queue>, max queue size=w825:i32, # elements in queue=w860:i32)  [unwired: 2 in, 5 out]
            n292 = Equal?(x=w860, y=0) -> (x = y?=w857:bool)
            n293 = Select(t=1, s=w799, f=w795) -> (s? t:f=w797:i32)
            n294 = Quotient & Remainder(x=w825, y=w824) -> (floor(x/y)=w823:i32)  [unwired: 1 out]
            n295 = case shown="True" w857 {
              tunnel: w856 -> [w931 w934]
              tunnel: w859 -> [w930 w935]
              tunnel: w823 -> [_ w936]
              tunnel: [w927 w933] -> w855
              tunnel: w858 -> [w929 w932]
              frame False {
                n296 = Lossy Enqueue Element(queue=w931, element=w930) -> (queue out=w928:refnum<queue>)  [unwired: 1 in, 3 out]
                n297 = Lossy Enqueue Element(queue=w928, element=w929) -> (queue out=w927:refnum<queue>)  [unwired: 1 in, 3 out]
              }
              frame True {
                n298 = for "For循环" {
                  N: w936 -> [_]
                  tunnel: w935 -> [w941]
                  tunnel: w934 -> [w940]
                  tunnel: [w938] -> w933
                  tunnel: w932 -> [w937]
                  n299 = Lossy Enqueue Element(queue=w940, element=w941) -> (queue out=w939:refnum<queue>)  [unwired: 1 in, 3 out]
                  n300 = Lossy Enqueue Element(queue=w939, element=w937) -> (queue out=w938:refnum<queue>)  [unwired: 1 in, 3 out]
                }
              }
            }
            n301 = Get Queue Status(queue=w855, return elements? (F)=w828) -> (queue out=w833:refnum<queue>, elements=w817:dbl[])  [unwired: 1 in, 6 out]
            n302 = local read "m(length of kernel)"() -> (w847:i32)
            n303 = local read "length of fish_history"() -> (w845:i32)
            n304 = feedback #6(w795) -> (w781:i32)
            n305 = Divide(x=1.0, y=30.0) -> (x/y=w842:dbl)
            n306 = expression code="atan(x)"(-0.043) -> (w841:dbl)
            n307 = Get Queue Status(queue=w852) -> (queue out=w851:refnum<queue>, max queue size=w827:i32, # elements in queue=w853:i32)  [unwired: 2 in, 5 out]
            n308 = Quotient & Remainder(x=w827, y=w824) -> (floor(x/y)=w826:i32)  [unwired: 1 out]
            n309 = Equal?(x=w853, y=0) -> (x = y?=w807:bool)
            n310 = case shown="True" w807 {
              tunnel: w851 -> [w916 w919]
              tunnel: w850 -> [w915 w920]
              tunnel: w826 -> [_ w921]
              tunnel: [w912 w918] -> w848
              tunnel: w849 -> [w914 w917]
              frame False {
                n311 = Lossy Enqueue Element(queue=w916, element=w915) -> (queue out=w913:refnum<queue>)  [unwired: 1 in, 3 out]
                n312 = Lossy Enqueue Element(queue=w913, element=w914) -> (queue out=w912:refnum<queue>)  [unwired: 1 in, 3 out]
              }
              frame True {
                n313 = for "For循环" {
                  N: w921 -> [_]
                  tunnel: w920 -> [w926]
                  tunnel: w919 -> [w925]
                  tunnel: [w922] -> w918
                  tunnel: w917 -> [w923]
                  n314 = Lossy Enqueue Element(queue=w925, element=w926) -> (queue out=w924:refnum<queue>)  [unwired: 1 in, 3 out]
                  n315 = Lossy Enqueue Element(queue=w924, element=w923) -> (queue out=w922:refnum<queue>)  [unwired: 1 in, 3 out]
                }
              }
            }
            n316 = Get Queue Status(queue=w848, return elements? (F)=w828) -> (queue out=w835:refnum<queue>, elements=w818:i32[])  [unwired: 1 in, 6 out]
            n317 = Max & Min(x=w783, y=w785) -> (max(x,y)=w794:i32)  [unwired: 1 out]
            n318 = Divide(x=w840, y=10000.0) -> (x/y=w837:dbl)
            n319 = Divide(x=w840, y=12800.0) -> (x/y=w836:dbl)
            n320 = feedback #7(w795) -> (w787:i32)
            n321 = case shown="True" "count" {
              tunnel: [w870 w872] -> w788
              tunnel: w787 -> [_ w871]
              tunnel: w781 -> [_ w872]
              tunnel: [w870 w871] -> w780
              frame False {
                w870 = 0
                "out of FOV 2" <- w870
                "max distance 2" <- w870
              }
              frame True {
                "out of FOV" <- w872
                "max distance" <- w871
              }
            }
            n322 = Add(x=w788, y=w797) -> (x+y=w796:i32)
            n323 = feedback-in #6(w796) -> ()
            n324 = Max & Min(x=w794, y=w780) -> (max(x,y)=w793:i32)  [unwired: 1 out]
            n325 = feedback-in #7(w793) -> ()
            n326 = Bundle(w815, w815) -> (w814:cluster{dbl, dbl})  [unwired: 1 in]
            n327 = dll-call lib="F:/TrackingUsingOpenCV3_with_bkg_subtr_and_pred_and_temp_matching_nodisplay - 210309/MPC_dll_4_vs17_cv3_4/x64/Release/MPC_dll_4_vs17_cv3_4.dll" fn="?MPC_dll@@YAHHHHNNNHNNNNNPEAV?$Point_@H@cv@@PEANPEAH21PEAV?$Point_@N@2@@Z"("m"=w847, "predict_length"=6 ("predict length"), "fish_history_length"=w845, "gammaX"="gamma", "gammaY"="gamma", "max_command"=10.0, "shift_head2yolk"="shift_head2yolk", "scale_x"=w842, "scale_y"=w842, "theta"=w841, "scale_x2"=w837, "scale_y2"=w836, "dst_fish_position"=w811, "command_history_array"=w819, "position_history_array"=w818, "fish_tr_history_c_array"=w829, "fish_direction_history_c_array"=w817, "c0"=w814) -> ("return type"=w779:i32, "c0"=w816:cluster{dbl, dbl})  [unwired: 20 in, 2 out]
            n328 = Equal To 0?(x=w779) -> (x = 0?=w777:bool)
            n329 = Not(x=w777) -> (.not. x?=w778:bool)
            n330 = case shown="False" w778 {
              tunnel: w810 -> [w899 w911]
              tunnel: w809 -> [w898 w910]
              tunnel: [w898 w909] -> w808
              tunnel: w806 -> [w900 w908]
              frame False {
                w888 = -inf
                n331 = local read "time loading a frame"() -> (w891:dbl)
                n332 = local read "TimeDelay"() -> (w893:dbl)
                n333 = call <vilib>:"High Resolution Relative Seconds.vi"() -> ("relative seconds"=w901:dbl)
                n334 = Not(x="reset 2") -> (.not. x?=w877:bool)
                n335 = Boolean To (0,1)(Boolean=w877) -> (0, 1=w876:i16)
                n336 = Subtract(x=w901, y=w899) -> (x-y=w878:dbl)
                n337 = Subtract(x=w900, y=w899) -> (x-y=w895:dbl)
                n338 = feedback #8(w888) -> (w897:dbl)
                n339 = feedback #9(w888) -> (w894:dbl)
                n340 = feedback #10(w888) -> (w896:dbl)
                n341 = Max & Min(x=w878, y=w897) -> (max(x,y)=w887:dbl)  [unwired: 1 out]
                "max time1 detection+command" <- w887
                n342 = feedback-in #8(w887) -> ()
                n343 = Max & Min(x=w893, y=w894) -> (max(x,y)=w890:dbl)  [unwired: 1 out]
                "max time3 total" <- w890
                n344 = feedback-in #9(w890) -> ()
                n345 = Max & Min(x=w895, y=w896) -> (max(x,y)=w875:dbl)  [unwired: 1 out]
                "max time2 detection" <- w875
                n346 = Multiply(x=w875, y=w876) -> (x*y=w874:dbl)
                n347 = feedback-in #10(w874) -> ()
                n348 = Greater?(x=w878, y=0.003) -> (0:w885:bool)
                n349 = feedback #11(w888) -> (w892:dbl)
                n350 = Select(t=1, s=w885, f=0) -> (s? t:f=w882:i32)
                n351 = Max & Min(x=w891, y=w892) -> (max(x,y)=w889:dbl)  [unwired: 1 out]
                "max time4 image and position loading" <- w889
                n352 = feedback-in #11(w889) -> ()
                n353 = feedback #12(0) -> (w881:i32)
                n354 = Add(x=w882, y=w881) -> (x+y=w880:i32)
                "#timeout1" <- w880
                n355 = feedback-in #12(w880) -> ()
              }
              frame True {
                n356 = call <vilib>:"High Resolution Relative Seconds.vi"() -> ("relative seconds"=w907:dbl)
                n357 = local read "TimeDelay"() -> (w905:dbl)
                n358 = local read "time loading a frame"() -> (w902:dbl)
                n359 = Subtract(x=w907, y=w911) -> (x-y=w906:dbl)
                n360 = Subtract(x=w908, y=w911) -> (x-y=w904:dbl)
                n361 = Format Into String(initial string=w910, w906, w904, w905, w902, "\r") -> (resulting string=w909:refnum<file>)  [unwired: 2 in, 1 out]
              }
            }
            n362 = Unbundle(w816) -> (w804:dbl, w805:dbl)
            n363 = Lossy Enqueue Element(queue=w831, element=w804) -> (queue out=w832:refnum<queue>)  [unwired: 1 in, 3 out]
            n364 = Lossy Enqueue Element(queue=w832, element=w805) -> (queue out=w830:refnum<queue>)  [unwired: 1 in, 3 out]
          }
        }
      }
      frame #3 {
      }
      frame #4 {
        n365 = Negate(x=w969) -> (-x=w968:dbl)
        "电压2" <- w968
        n366 = call-poly <vilib>:"DAQmx Write.vi"("task/channels in"=w972, "data"=w970) -> ("task out"=w973:refnum<k21>)  [unwired: 11 in, 2 out]
        n367 = call-poly <vilib>:"DAQmx Write.vi"("task/channels in"=w971, "data"=w968) -> ("task out"=w974:refnum<k21>)  [unwired: 11 in, 2 out]
        "电压1" <- w970
      }
      frame #5 {
        n368 = call <vilib>:"High Resolution Relative Seconds.vi"() -> ("relative seconds"=w984:dbl)
      }
    }
    n369 = flat-sequence {
      tunnel: w361 -> [w998]
      tunnel: [w996] -> w468
      frame #0 {
        n370 = Unbundle By Name(w998) -> ("status"=w999:bool)
        n371 = local read "Stopped"() -> (w997:bool)
        n372 = Compound Arithmetic op=OR(w999, "Stop", w997) -> (w996:bool)
        n373 = local write "Stopped"(w996) -> ()
      }
    }
    n374 = feedback-in #13(w468) -> ()
    n375 = feedback #13() -> (w467:bool)  [unwired: 1 in]
    n376 = node-c288() -> ()  [unwired: 1 in, 1 out]
  }
  n377 = Close File(refnum=w45) -> ()  [unwired: 1 in, 2 out]
  n378 = call-poly <vilib>:"DAQmx Write.vi"("task/channels in"=w97, "data"=0.0) -> ("task out"=w95:refnum<k21>)  [unwired: 11 in, 2 out]
  n379 = call <vilib>:"DAQmx Stop Task.vi"("task/channels in"=w95) -> ("task out"=w91:refnum<k21>)  [unwired: 13 in, 1 out]
  n380 = call-poly <vilib>:"DAQmx Write.vi"("task/channels in"=w96, "data"=0.0) -> ("task out"=w93:refnum<k21>)  [unwired: 11 in, 2 out]
  n381 = call <vilib>:"DAQmx Stop Task.vi"("task/channels in"=w93) -> ("task out"=w90:refnum<k21>)  [unwired: 13 in, 1 out]
  n382 = call <vilib>:"DAQmx Clear Task.vi"("task in"=w91) -> ()  [unwired: 14 in, 1 out]
  n383 = call <vilib>:"DAQmx Clear Task.vi"("task in"=w90) -> ()  [unwired: 14 in, 1 out]
  n384 = node-c288(w31) -> ()  [unwired: 1 out]
  n385 = Release Queue(queue=w52) -> ()  [unwired: 2 in, 3 out]
  n386 = Release Queue(queue=w51) -> ()  [unwired: 2 in, 3 out]
  n387 = Release Queue(queue=w50) -> ()  [unwired: 2 in, 3 out]
  n388 = Release Queue(queue=w49) -> ()  [unwired: 2 in, 3 out]
  n389 = call <userlib>:"DAQNavi Stop Task.vi"("task in"=w73) -> ("task out"=w75:i32)  [unwired: 1 in, 1 out]
  n390 = Merge Errors(w130, w129) -> (w131:errorcluster)
  n391 = call <userlib>:"DAQNavi Stop Task.vi"("task in"=w72) -> ("task out"=w74:i32)  [unwired: 1 in, 1 out]
  n392 = flat-sequence {
    tunnel: w131 -> [w1002]
    tunnel: [w1002] -> w138
    tunnel: w137 -> [w1003]
    tunnel: w24 -> [_]
    frame #0 {
      n393 = local write "Initialized"(FALSE ("Module Enabled")) -> ()
      n394 = call "IMAQ Dispose"("Image"=w1003) -> ()  [unwired: 5 in, 1 out]
    }
  }
  n395 = call <userlib>:"DAQNavi Clear Task.vi"("task in"=w75) -> ()  [unwired: 2 in, 1 out]
  n396 = call <userlib>:"DAQNavi Clear Task.vi"("task in"=w74) -> ()  [unwired: 2 in, 1 out]
  n397 = xnode "关闭FPGA VI引用"("FPGA VI引用输入"=w139, "错误输入"=w138) -> ("错误输出"=w136:errorcluster)
  n398 = call <vilib>:"Simple Error Handler.vi"("error in (no error)"=w136) -> ()  [unwired: 4 in, 5 out]
